vi "menu-Cal group disabled state.vi"(8 "error in (no error)":errorcluster) -> (0 "error out":errorcluster, 3 "menu reference out":refnum<k9>)   [LabVIEW 2013]
uses:
  Global Variables/gl_UI Ctrl Refs.vi
  Global Variables/General Globals.vi
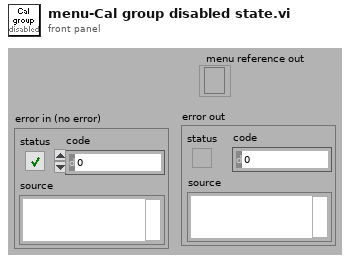
[diagram p1: front panel]
types:
  T1 = typedef "UI ctrl refs cluster.ctl" = cluster{"Top level VI path":path, "Top level VI ref":refnum<vi>, "User menu ref":refnum<k9>, "Sub Panel control":refnum<vi>, "Imaging Param Tab":refnum<vi>, "Occurrence-Start drivers":refnum<k4>, "Occurrence-Speed logging initialised":refnum<k4>, "Occurrence-XYZ stage initialised":refnum<k4>, "Exit button":refnum<vi>, "Status ind":refnum<vi>, "Return to Origin":refnum<vi>, "Speed Logging":refnum<vi>, "Time Lapse":refnum<vi>, "Live Imaging":refnum<vi>, "AOL Z Stack":refnum<vi>, "Motor Z Stack":refnum<vi>, "Funct Acq button":refnum<vi>, "Hard Shutter":refnum<vi>, "Virtual Shutter":refnum<vi>, "Laser Power":refnum<vi>, "AOL Mode":refnum<vi>, "Frame Size":refnum<vi>, "Field of View":refnum<vi>, "Dwell Time":refnum<vi>, "Zoom":refnum<vi>, "AOL Z":refnum<vi>, "Objective":refnum<vi>, "Axis":refnum<vi>, "Paths & Names":refnum<vi>, "Experiment folder path (ind.)":refnum<vi>, "Last State (Ind.)":refnum<vi>, "Laser wavelength ind (nm)":refnum<vi>, "Averages":refnum<vi>, "Angle (degrees)":refnum<vi>, "X centre":refnum<vi>, "Y centre":refnum<vi>, "Plane Mode":refnum<vi>, "# Planes":refnum<vi>, "Z Start":refnum<vi>, "Z Stop":refnum<vi>, "Z Step":refnum<vi>, "PMT 1":refnum<vi>, "PMT 2":refnum<vi>, "Stage XYZ Position":refnum<vi>, "Pockels@Z Start":refnum<vi>, "Pockels@Z Stop":refnum<vi>, "Obtain Z Start":refnum<vi>, "Obtain Z Stop":refnum<vi>, "Live stim.trig.period":refnum<vi>, "Live stim.trig.enable":refnum<vi>, "Funct. Acq. Pockels Modulation":refnum<vi>, "Enable Video Recording":refnum<vi>, "Video Record-Live Imaging":refnum<vi>, "Video Record-Funct acq":refnum<vi>, "AOL Z-stack Chirps Ready (ind)":refnum<vi>, "Center freq ind (nm)":refnum<vi>, "Logging queue (ind)":refnum<vi>, "Back aperture power (ind.)":refnum<vi>, "Power after objective (ind.)":refnum<vi>, "Switch user":refnum<vi>}
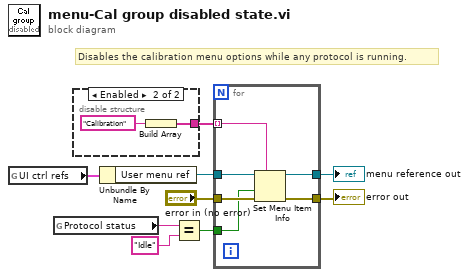
[diagram p0: block diagram]
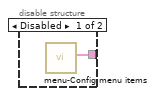
[diagram p2: hidden frame]
diagram:
  # "Disables the calibration menu options while any protocol is running."
  n1 = global read "gl_UI Ctrl Refs.vi" "UI ctrl refs"() -> (w9:T1)
  n2 = global read "General Globals.vi" "Protocol status"() -> (w1:string)
  n3 = disable-structure shown="Enabled" {
    disable-tunnel: [w10 w11] -> w4
    frame Disabled {
      n4 = call "menu-Config menu items.vi"() -> ("item tags"=w10:string[])  [unwired: 10 in, 1 out]
    }
    frame Enabled {
      n5 = Build Array("Calibration") -> (w11:string[])
    }
  }
  n6 = Unbundle By Name(w9) -> ("User menu ref"=w6:refnum<k9>)
  n7 = Equal?(x=w1, y="Idle") -> (x = y?=w2:bool)
  n8 = for {
    tunnel: [w18] -> w8
    tunnel: [w17] -> w7
    tunnel: w6 -> [w16]
    tunnel: "error in (no error)" -> [w15]
    tunnel: w4 -> [w14] mode=indexing
    tunnel: w2 -> [w13]
    n9 = Set Menu Item Info(7:w14, 8:w15, 9:w13, 11:w16) -> (0:w17:errorcluster, 3:w18:refnum<k9>)  [unwired: 1 in, 2 out]
  }
  "error out" <- w7
  "menu reference out" <- w8
